vi "RangeAndSetupQDC.vi"(6 "Count only accepted trigs?\n(else all trigs)":bool, 7 "VME module Base Address":u32, 8 "error in (no error)":errorcluster, 9 "High range threshold":u16, 10 "handle in":i32, 11 "Low Range threshold":u16) -> (0 "error out":errorcluster, 3 "handle out":i32)   [LabVIEW 2014]
uses:
  Program Files (x86)/CAEN/Comm/labview/CAENComm.lvlib
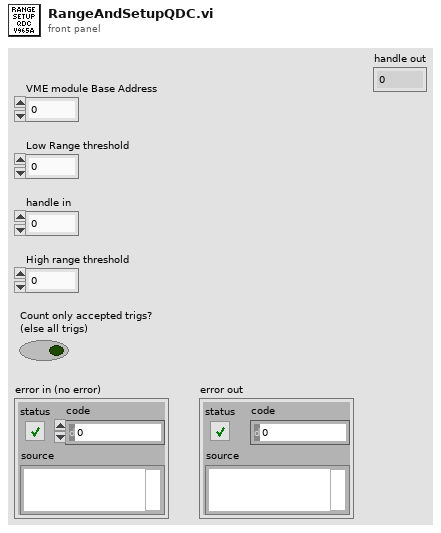
[diagram p1: front panel]
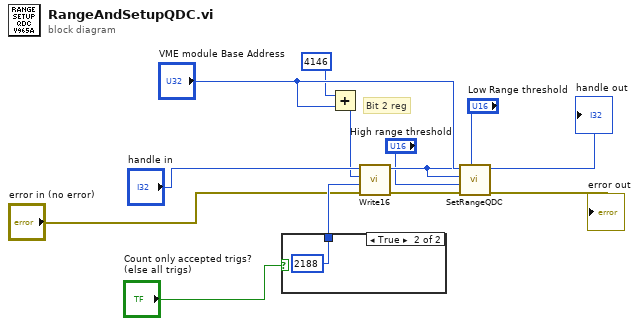
[diagram p0: block diagram]
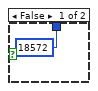
[diagram p2: hidden frame]
diagram:
  # "Bit 2 reg"
  n1 = case shown="True" "Count only accepted trigs?\n(else all trigs)" {
    tunnel: [18572 2188] -> w5
    frame False {
    }
    frame True {
    }
  }
  n2 = Add(x=u32 4146, y="VME module Base Address") -> (x+y=w3:u32)
  n3 = call "Write16.vi"("error in (no error)"="error in (no error)", "Data"=w5, "Address"=w3, "handle"="handle in") -> ("error out"=w6:errorcluster)  [unwired: 7 in]
  n4 = call "SetRangeQDC.vi"("Low Range threshold"="Low Range threshold", "error in (no error)"=w6, "High range threshold"="High range threshold", "handle"="handle in", "VME module Base Address"="VME module Base Address") -> ("error out"=→"error out":errorcluster)  [unwired: 6 in]
  "handle out" <- "handle in"
